vi "take-picture.vi"(8 "factor":dbl, 10 "path to JPEG file":path) -> (2 "new picture":picture)   [LabVIEW 2014]
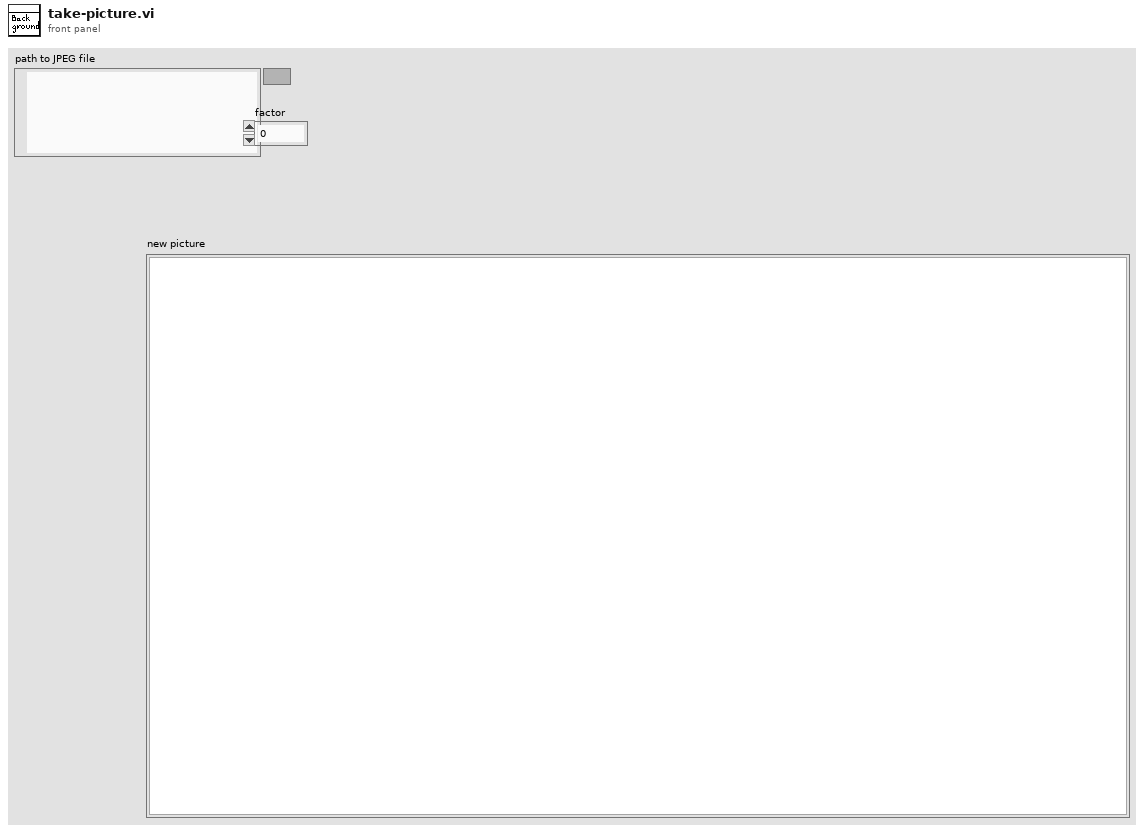
[diagram p1: front panel]
types:
  T1 = typedef "LVBoundsTypeDef.ctl" = cluster{"Width":u32, "Height":u32}
  T2 = typedef "imagedata.ctl" = cluster{"image type":i32, "image depth":i32, "image":u8[], "mask":u8[], "colors":u32[], "Rectangle":cluster{"left":i16, "top":i16, "right":i16, "bottom":i16}}
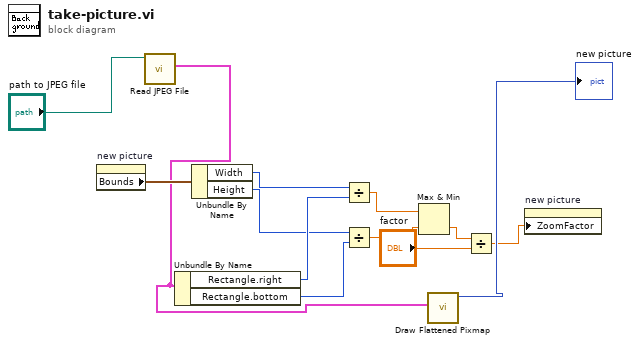
[diagram p0: block diagram]
diagram:
  n1 = property on="new picture" class="Pict"() -> ("Bounds"=w12:T1)  [unwired: 2 in, 2 out]
  n2 = call <vilib>:"Read JPEG File.vi"("path to JPEG file"="path to JPEG file") -> ("image data"=w5:T2)  [unwired: 8 in, 2 out]
  n3 = Unbundle By Name(w5) -> ("Rectangle.right"=w10:i16, "Rectangle.bottom"=w8:i16)
  n4 = Unbundle By Name(w12) -> ("Width"=w11:u32, "Height"=w9:u32)
  n5 = Divide(x=w11, y=w10) -> (x/y=w7:dbl)
  n6 = Divide(x=w9, y=w8) -> (x/y=w6:dbl)
  n7 = Max & Min(x=w7, y=w6) -> (min(x,y)=w3:dbl)  [unwired: 1 out]
  n8 = call <vilib>:"Draw Flattened Pixmap.vi"("image data"=w5) -> ("new picture"=→"new picture":picture)  [unwired: 8 in]
  n9 = Divide(x=w3, y="factor") -> (x/y=w2:dbl)
  n10 = property on="new picture" class="Pict"("ZoomFactor"=w2) -> ()  [unwired: 2 in, 2 out]
